vi "Create Log File.vi"(8 "error in (no error)":errorcluster, 10 "log file name":string, 11 "log file directory":path) -> (0 "error out":errorcluster, 3 "file refnum":refnum<file>)   [LabVIEW 2021, in "DSF Core.lvlib" / "Logging Thread.lvclass"]
uses:
  Logging Thread.lvclass
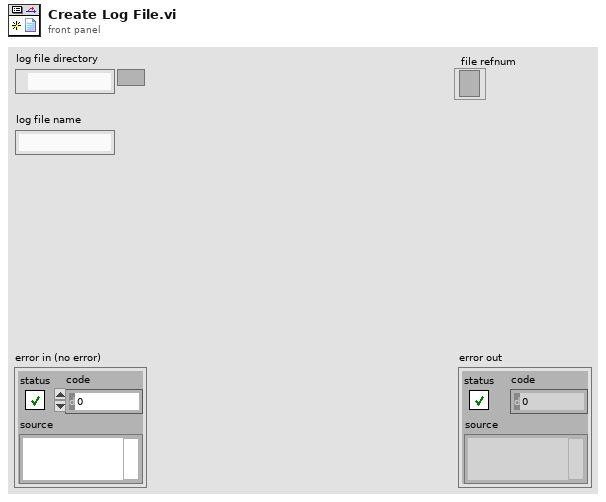
[diagram p1: front panel]
types:
  T1 = enum16{"open", "replace", "create", "open or create", "replace or create", "replace or create with confirmation"}
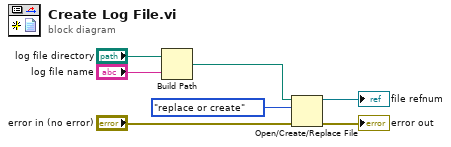
[diagram p0: block diagram]
diagram:
  n1 = Build Path(base path="log file directory", name or relative path="log file name") -> (appended path=w2:path)
  n2 = Open/Create/Replace File(file path (use dialog)=w2, error in="error in (no error)", operation (0:open)=T1."replace or create") -> (refnum out=→"file refnum":refnum<file>, error out=→"error out":errorcluster)  [unwired: 3 in, 1 out]
